vi "StartModsICDAS.vi"(6 "Visualization VI Paths":path[](array[path]), 7 "ShowPanel? (f)":bool=TRUE, 8 "Error Array In":errorcluster[](array[cluster]), 9 "INI File Paths":path[](array[path]), 10 "Module List":string[](array[string]), 11 "Test.lvclass":refnum<class "Test.lvclass">) -> (0 "Error Array Out":errorcluster[](array[cluster]), 2 "Event Array":variant[](array[variant]), 3 "Test.lvclass":refnum<class "Test.lvclass">)   [LabVIEW 2018]
doc: "Instantiates a module based on the module list."
uses:
  NistPluggableModules/TestClass/Test.lvclass
  NistPluggableModules/TestClass/Test.lvclass/Test.ctl
  NistPluggableModules/TestClass/Accessors/Read ModuleList.vi
  NistPluggableModules/TestClass/Accessors/Read ModuleIDs.vi
  NistPluggableModules/TestClass/Accessors/Read CloneReg.vi
  NistPluggableModules/TestClass/Accessors/Write ModuleList.vi
  NistPluggableModules/TestClass/Accessors/Write ModuleIDs.vi
  NistPluggableModules/TestClass/Accessors/Write CloneReg.vi
  <userlib>/NIST/ModuleAdminLib/CloneRegistration/CloneRegistration.lvclass
  <userlib>/NIST/NISTErrorLib/NISTErrorLib.lvlib
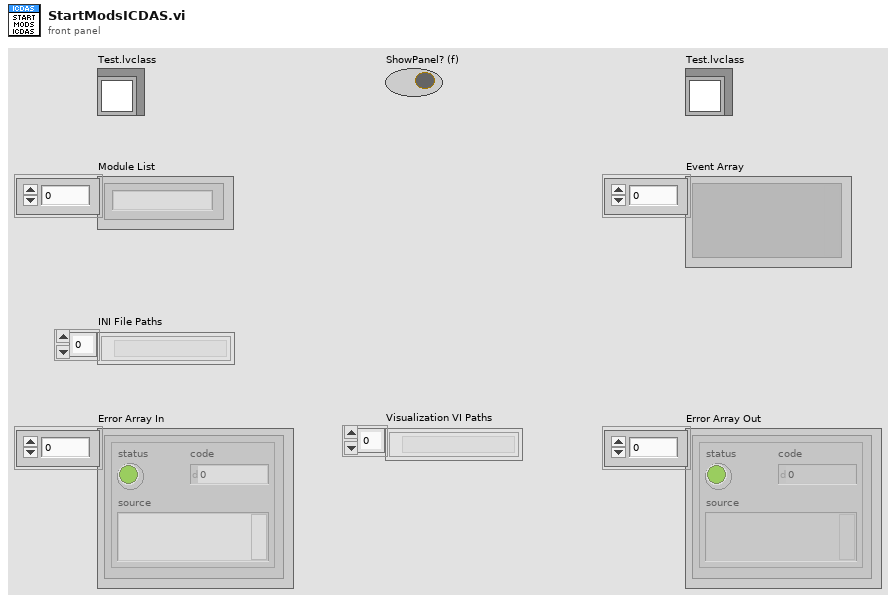
[diagram p1: front panel]
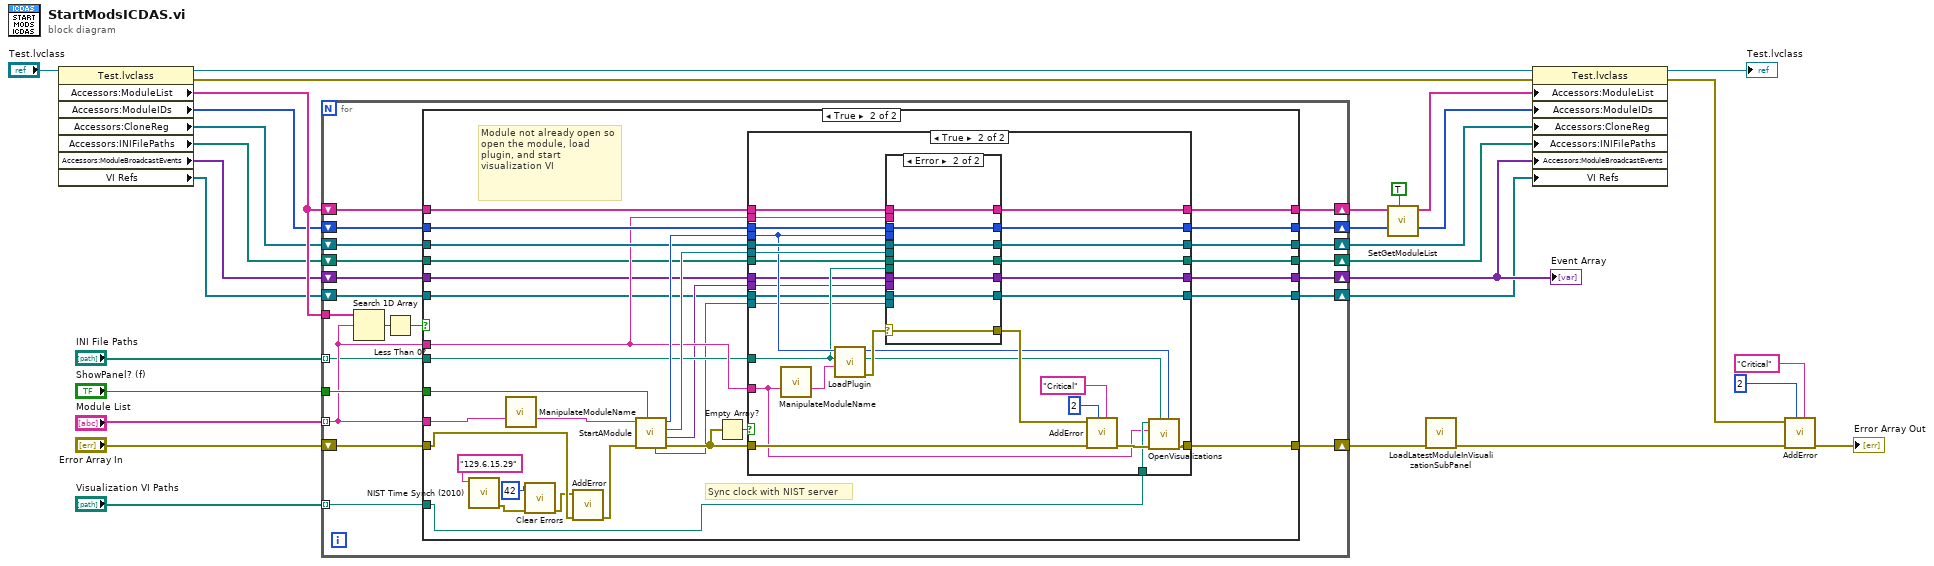
[diagram p0: block diagram]
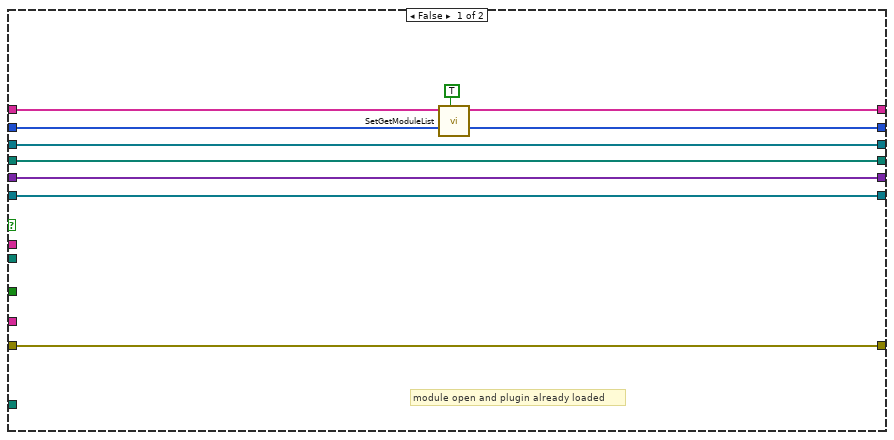
[diagram p2: hidden frame]
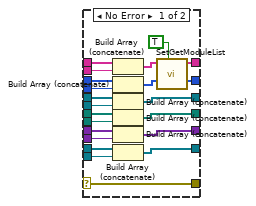
[diagram p4: hidden frame]
diagram:
  n1 = property class="Test.lvclass"(reference="Test.lvclass") -> (reference out=w20:refnum<class "Test.lvclass">, error out=w19:errorcluster, "Accessors:ModuleList"=w18:string[], "Accessors:ModuleIDs"=w17:i32[], "Accessors:CloneReg"=w16:refnum<data-value>[], "Accessors:INIFilePaths"=w8:path[], "Accessors:ModuleBroadcastEvents"=w6:variant[], "VI Refs"=w2:refnum<vi>[])  [unwired: 1 in]
  n2 = for {
    tunnel: "ShowPanel? (f)" -> [w50]
    tunnel: "Module List" -> [w43] mode=indexing
    shift-right: [w49] -> w4
    shift-left: "Error Array In" -> [w48]
    tunnel: w18 -> [w47]
    shift-right: [w38] -> w15
    shift-left: w18 -> [w44]
    shift-right: [w40] -> w14
    shift-left: w17 -> [w42]
    shift-right: [w39] -> w13
    shift-left: w16 -> [w41]
    tunnel: "INI File Paths" -> [w37] mode=indexing
    tunnel: "Visualization VI Paths" -> [w36] mode=indexing
    shift-right: [w34] -> w7
    shift-left: w8 -> [w35]
    shift-right: [w32] -> w5
    shift-left: w6 -> [w33]
    shift-right: [w30] -> w1
    shift-left: w2 -> [w31]
    n3 = Search 1D Array(1D array=w47, element=w43) -> (index of element=w46:i32)  [unwired: 1 in]
    n4 = Less Than 0?(x=w46) -> (x < 0?=w45:bool)
    n5 = case shown="True" w45 {
      tunnel: w50 -> [_ w73]
      tunnel: [w56 w76] -> w49
      tunnel: w43 -> [_ w90]
      tunnel: w48 -> [w56 w64]
      tunnel: w44 -> [w59 w88]
      tunnel: w43 -> [_ w79]
      tunnel: w42 -> [w58 w87]
      tunnel: w41 -> [w57 w85]
      tunnel: [w58 w83] -> w40
      tunnel: [w57 w82] -> w39
      tunnel: [w53 w81] -> w38
      tunnel: w37 -> [_ w78]
      tunnel: w36 -> [_ w66]
      tunnel: w35 -> [w55 w75]
      tunnel: [w55 w74] -> w34
      tunnel: w33 -> [w54 w72]
      tunnel: [w54 w70] -> w32
      tunnel: w31 -> [w51 w69]
      tunnel: [w51 w67] -> w30
      frame False {
        # "module open and plugin already loaded"
        n6 = call "SetGetModuleList.vi"("Set? (F)"=TRUE, "ModuleList"=w59) -> ("ModuleList"=w53:string[])  [unwired: 9 in]
      }
      frame True {
        # "Sync clock with NIST server"
        # "Module not already open so open the module, load plugin, and start visualization VI"
        n7 = call "NIST Time Synch (2010).vi"("Time Server IP Address (129.6.15.29)"="129.6.15.29") -> ("error out"=w63:errorcluster)  [unwired: 6 in]
        n8 = call "ManipulateModuleName.vi"("ModuleListSingleEntry"=w90) -> ("BeforeMatch:ModuleListSingleEntry"=w89:string)  [unwired: 9 in, 5 out]
        n9 = call <vilib>:"Clear Errors.vi"("error in (no error)"=w63, "specific error code to clear (0: all)"=42) -> ("error out"=w60:errorcluster)  [unwired: 4 in, 1 out]
        n10 = call <userlib>:"AddError.vi"("ErrorArray In"=w64, "error in (no error)"=w60) -> ("ErrorArray Out"=w65:errorcluster[])  [unwired: 8 in, 1 out]
        n11 = call "StartAModule.vi"("ShowPanel?"=w73, "Error Array In"=w65, "Module Name (Sensor, Fgen, etc.)"=w89) -> ("ErrorArray Out"=w77:errorcluster[], "Variant"=w71:variant, "Clone Registration"=w84:refnum<data-value>, "Module ID"=w86:i32, "VI Ref"=w68:refnum<vi>)  [unwired: 4 in]
        n12 = Empty Array?(array=w77) -> (empty?=w80:bool)
        n13 = case shown="True" w80 {
          tunnel: w88 -> [w97 w127]
          tunnel: w79 -> [_ w126]
          tunnel: w87 -> [w95 w125]
          tunnel: w86 -> [_ w119]
          tunnel: w85 -> [w96 w124]
          tunnel: w84 -> [_ w123]
          tunnel: [w95 w122] -> w83
          tunnel: [w96 w121] -> w82
          tunnel: [w97 w111] -> w81
          tunnel: w79 -> [_ w112]
          tunnel: w78 -> [_ w107]
          tunnel: w77 -> [w94 w116]
          tunnel: w66 -> [_ w114]
          tunnel: [w94 w113] -> w76
          tunnel: w75 -> [w93 w108]
          tunnel: [w93 w106] -> w74
          tunnel: w72 -> [w92 w105]
          tunnel: w71 -> [_ w104]
          tunnel: [w92 w103] -> w70
          tunnel: w69 -> [w91 w100]
          tunnel: w68 -> [_ w99]
          tunnel: [w91 w98] -> w67
          frame False {
          }
          frame True {
            n14 = call "ManipulateModuleName.vi"("ModuleListSingleEntry"=w112) -> ("BeforeMatch:ModuleListSingleEntry"=w120:string)  [unwired: 9 in, 5 out]
            n15 = call "LoadPlugin.vi"("Module Name"=w120, "INI File Path"=w107, "Module ID"=w119) -> ("error out"=w110:errorcluster, "INI File Path out"=w101:path, "Module ID out"=w102:i32)  [unwired: 5 in, 1 out]
            n16 = case shown="Error" w110 {
              selector: w110 -> [w137 w152]
              tunnel: w127 -> [w148 w155]
              tunnel: w126 -> [w147 _]
              tunnel: w125 -> [w146 w154]
              tunnel: w124 -> [w145 w153]
              tunnel: w123 -> [w144 _]
              tunnel: [w143 w154] -> w122
              tunnel: [w142 w153] -> w121
              tunnel: w119 -> [w141 _]
              tunnel: [w139 w155] -> w111
              tunnel: [w137 w152] -> w109
              tunnel: w108 -> [w136 w151]
              tunnel: w107 -> [w135 _]
              tunnel: [w134 w151] -> w106
              tunnel: w105 -> [w133 w150]
              tunnel: w104 -> [w132 _]
              tunnel: [w131 w150] -> w103
              tunnel: w100 -> [w130 w149]
              tunnel: w99 -> [w129 _]
              tunnel: [w128 w149] -> w98
              frame No Error {
                n17 = Build Array (concatenate)(w148, w147) -> (w140:string[])
                n18 = Build Array (concatenate)(w146, w141) -> (w143:i32[])
                n19 = Build Array (concatenate)(w145, w144) -> (w142:refnum<data-value>[])
                n20 = Build Array (concatenate)(w136, w135) -> (w134:path[])
                n21 = Build Array (concatenate)(w133, w132) -> (w131:variant[])
                n22 = Build Array (concatenate)(w130, w129) -> (w128:refnum<vi>[])
                n23 = call "SetGetModuleList.vi"("Set? (F)"=TRUE, "ModuleList"=w140) -> ("ModuleList"=w139:string[])  [unwired: 9 in]
              }
              frame Error {
              }
            }
            n24 = call <userlib>:"AddError.vi"("Severity"="Critical", "Priority"=u8 2, "ErrorArray In"=w116, "error in (no error)"=w109) -> ("ErrorArray Out"=w115:errorcluster[])  [unwired: 6 in, 1 out]
            n25 = call "OpenVisualizations.vi"("ModuleID"=w102, "INIFilePath"=w101, "ErrorArray in"=w115, "Module Name (e.g. Sensor.RoomAlert.Model-4E)"=w112, "Visualization VI Path"=w114) -> ("ErrorArray out"=w113:errorcluster[])  [unwired: 6 in]
          }
        }
      }
    }
  }
  "Event Array" <- w5
  n26 = call "SetGetModuleList.vi"("Set? (F)"=TRUE, "ModuleList"=w15) -> ("ModuleList"=w10:string[])  [unwired: 9 in]
  n27 = call "LoadLatestModuleInVisualizationSubPanel.vi"("Error Array In in"=w4) -> ("Error Array In out"=w3:errorcluster[])  [unwired: 10 in]
  n28 = property class="Test.lvclass"(reference=w20, error in=w19, "Accessors:ModuleList"=w10, "Accessors:ModuleIDs"=w14, "Accessors:CloneReg"=w13, "Accessors:INIFilePaths"=w7, "Accessors:ModuleBroadcastEvents"=w5, "VI Refs"=w1) -> (reference out=→"Test.lvclass":refnum<class "Test.lvclass">, error out=w25:errorcluster)
  n29 = call <userlib>:"AddError.vi"("Severity"="Critical", "Priority"=u8 2, "ErrorArray In"=w3, "error in (no error)"=w25) -> ("ErrorArray Out"=→"Error Array Out":errorcluster[])  [unwired: 6 in, 1 out]
